vi "example_2_7_a.vi"() -> ()   [LabVIEW 2018]
panel:
  in  "stop":bool
  in  "START_BUTTON":bool
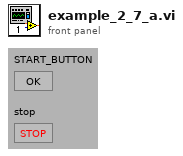
[diagram p1: front panel]
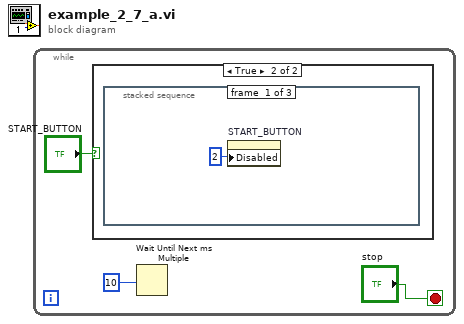
[diagram p0: block diagram]
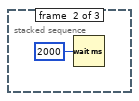
[diagram p3: hidden frame]
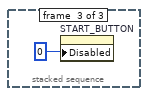
[diagram p4: hidden frame]
diagram:
  n1 = while {
    stop <- "stop" stop-if-true
    n2 = case shown="True" "START_BUTTON" {
      frame False {
      }
      frame True {
        n3 = stacked-sequence {
          frame #0 {
            n4 = property on="START_BUTTON" class="Bool"("Disabled"=u8 2) -> ()  [unwired: 2 in, 2 out]
          }
          frame #1 {
            n5 = Wait (ms)(milliseconds to wait=u32 2000) -> ()  [unwired: 1 out]
          }
          frame #2 {
            n6 = property on="START_BUTTON" class="Bool"("Disabled"=u8 0) -> ()  [unwired: 2 in, 2 out]
          }
        }
      }
    }
    n7 = Wait Until Next ms Multiple(millisecond multiple=u32 10 ("milliseconds to wait")) -> ()  [unwired: 1 out]
  }
